vi "HexStringArrayToByteArray.vi"(5 "HexStirngArray":string="00 0A 0B 0C 0D FF") -> (2 "ByteArrayOut":u8[](array[numeric]) format="%02x")   [LabVIEW 2011, in "GenericCanAdapterClass.lvclass"]
uses:
  GenericCanAdapterClass.lvclass
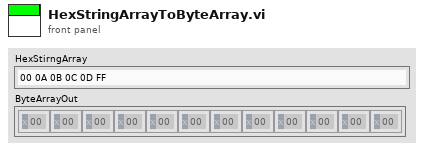
[diagram p1: front panel]
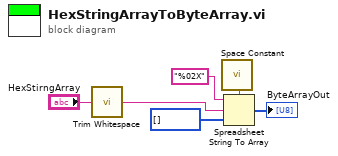
[diagram p0: block diagram]
diagram:
  n1 = call <vilib>:"Trim Whitespace.vi"("string"="HexStirngArray") -> ("trimmed string"=w6:string)  [unwired: 1 in]
  n2 = call <vilib>:"Space Constant.vi"() -> ("String"=w5:string)
  n3 = Spreadsheet String To Array(delimiter (Tab)=w5, format string="%02X", spreadsheet string=w6, array type (2D Dbl)=u8[] [] ("Response")) -> (array=→"ByteArrayOut":u8[])
